vi "HIOKI PW3390 Conf Current.vi"(0 "VISA Resource":refnum<visa-resource-name>, 1 "Set/Query (F: Set)":bool, 2 "CH (1)":i32=1 min=1 max=4, 5 "Auto (F: OFF)":bool, 7 "Range (18: 500A)":T1(ring)=enum."500", 9 "I rect (F: RMS)":bool, 11 "error in (no error)":errorcluster, 12 "OPC query (T: ON)":bool=TRUE, 13 "Error Out (F: Off)":bool) -> (4 "VISA Resource out":refnum<visa-resource-name>, 6 "Auto out":bool, 8 "Range out":dbl=500.0 format="%.1f", 10 "I rect out":bool, 15 "error out":errorcluster)   [LabVIEW 2009]
doc: "Set/Query\n Set: Send the setting commands for the device.\n Query: Query the setting of the device.\n\nAuto\n Sets the current range to AutoRange.\n\nRange\n Sets the current range. Valid when the AutoRange is OFF.\n\nI rect\n Sets the Electric Current Rectification Method to RMS/MEAN.\n\n<B>Note</B>\n Depending on the measurement line combination (for 1P3W and above), the current AutoRange settings of other channels in the combination may be changed too."
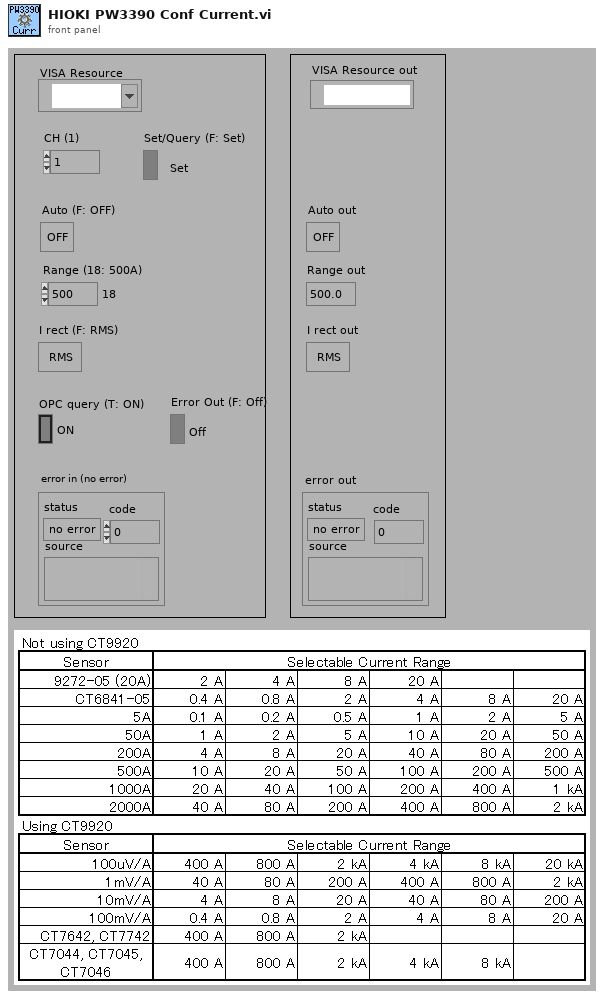
[diagram p1: front panel]
types:
  T1 = enum16{"0.1", "0.2", "0.4", "0.5", "0.8", "1", "2", "4", "5", "8", "10", "20", "40", "50", "80", "100", "200", "400", "500", "800", "1000", "2000", "4000", "8000", "20000"}
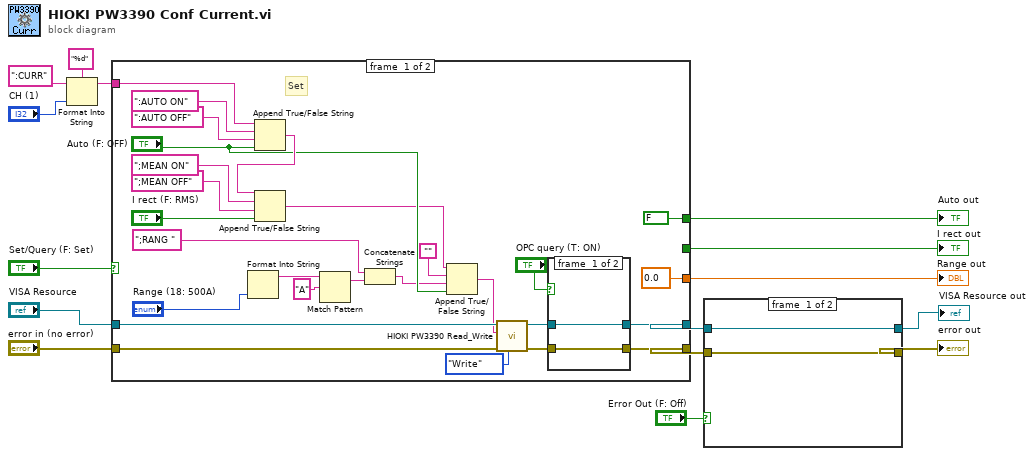
[diagram p0: block diagram]
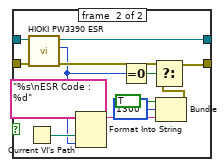
[diagram p2: hidden frame]
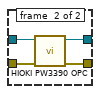
[diagram p3: hidden frame]
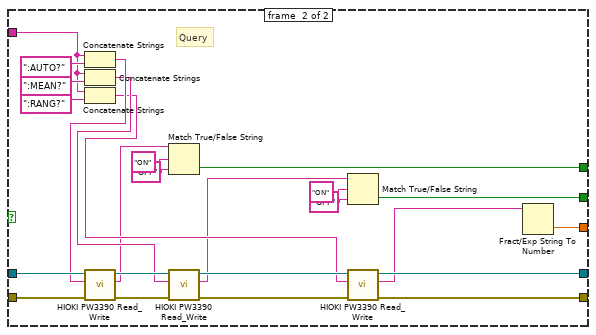
[diagram p4: hidden frame]
diagram:
  n1 = Format Into String(format string="%d", initial string=":CURR", "CH (1)") -> (resulting string=w10:string)  [unwired: 1 in, 1 out]
  n2 = case shown="FALSE" "Set/Query (F: Set)" {
    tunnel: "error in (no error)" -> [w29 w57]
    tunnel: [w22 w56] -> w5
    tunnel: "VISA Resource" -> [w30 w58]
    tunnel: [w23 w55] -> w4
    tunnel: w10 -> [w38 w69]
    tunnel: [0.0 w72] -> w9
    tunnel: [w41 w64] -> w8
    tunnel: [w41 w63] -> w7
    frame #0 {
      w41 = FALSE
      # "Set"
      n3 = Format Into String("Range (18: 500A)") -> (resulting string=w21:string)  [unwired: 3 in, 1 out]
      n4 = Append True/False String(1:"Auto (F: OFF)", 2:":AUTO OFF", 3:":AUTO ON", 4:w38) -> (0:w34:string)
      n5 = Append True/False String(1:"I rect (F: RMS)", 2:";MEAN OFF", 3:";MEAN ON", 4:w34) -> (0:w32:string)
      n6 = Match Pattern(string=w21, regular expression="A") -> (before substring=w18:string)  [unwired: 1 in, 3 out]
      n7 = Concatenate Strings(";RANG ", w18) -> (w16:string)
      n8 = Append True/False String(1:"Auto (F: OFF)", 2:w16, 3:"", 4:w32) -> (0:w28:string)
      n9 = call <instrlib>:"HIOKI PW3390 Read_Write.vi"("Read/Write"=enum16{"Read", "Write"}."Write", "error in (no error)"=w29, "data in"=w28, "VISA Resource"=w30) -> ("error out"=w24:errorcluster, "VISA Resource out"=w25:refnum<visa-resource-name>)  [unwired: 5 in, 1 out]
      n10 = case shown="TRUE" "OPC query (T: ON)" {
        tunnel: [w44 w48] -> w23
        tunnel: [w43 w47] -> w22
        tunnel: w25 -> [w44 w46]
        tunnel: w24 -> [w43 w45]
        frame #0 {
        }
        frame #1 {
          n11 = call <instrlib>:"HIOKI PW3390 OPC.vi"("error in (no error)"=w45, "VISA Resource"=w46) -> ("error out"=w47:errorcluster, "VISA Resource out"=w48:refnum<visa-resource-name>)  [unwired: 7 in, 1 out]
        }
      }
    }
    frame #1 {
      # "Query"
      n12 = Concatenate Strings(w69, ":AUTO?") -> (w54:string)
      n13 = Concatenate Strings(w69, ":MEAN?") -> (w53:string)
      n14 = Concatenate Strings(w69, ":RANG?") -> (w52:string)
      n15 = call <instrlib>:"HIOKI PW3390 Read_Write.vi"("error in (no error)"=w57, "data in"=w54, "VISA Resource"=w58) -> ("error out"=w61:errorcluster, "data out"=w51:string, "VISA Resource out"=w59:refnum<visa-resource-name>)  [unwired: 6 in]
      n16 = Match True/False String(2:"OFF", 3:"ON", 4:w51) -> (0:w64:bool)  [unwired: 1 out]
      n17 = call <instrlib>:"HIOKI PW3390 Read_Write.vi"("error in (no error)"=w61, "data in"=w53, "VISA Resource"=w59) -> ("error out"=w62:errorcluster, "data out"=w50:string, "VISA Resource out"=w60:refnum<visa-resource-name>)  [unwired: 6 in]
      n18 = Match True/False String(2:"OFF", 3:"ON", 4:w50) -> (0:w63:bool)  [unwired: 1 out]
      n19 = call <instrlib>:"HIOKI PW3390 Read_Write.vi"("error in (no error)"=w62, "data in"=w52, "VISA Resource"=w60) -> ("error out"=w56:errorcluster, "data out"=w49:string, "VISA Resource out"=w55:refnum<visa-resource-name>)  [unwired: 6 in]
      n20 = Fract/Exp String To Number(string=w49) -> (number=w72:dbl)  [unwired: 3 in, 1 out]
    }
  }
  "Auto out" <- w8
  "I rect out" <- w7
  "Range out" <- w9
  n21 = case shown="TRUE" "Error Out (F: Off)" {
    tunnel: w4 -> [w75 w88]
    tunnel: w5 -> [w74 w87]
    tunnel: [w74 w77] -> w3
    tunnel: [w75 w86] -> w1
    frame #0 {
    }
    frame #1 {
      n22 = Current VI's Path() -> (path=w84:path)
      n23 = call <instrlib>:"HIOKI PW3390 ESR.vi"("error in (no error)"=w87, "VISA Resource"=w88) -> ("error out"=w78:errorcluster, "Output Value"=w76:u8, "VISA Resource out"=w86:refnum<visa-resource-name>)  [unwired: 6 in, 1 out]
      n24 = Format Into String(format string="%s\nESR Code : %d", w84, w76) -> (resulting string=w80:string)  [unwired: 2 in, 1 out]
      n25 = Equal To 0?(x=w76) -> (x = 0?=w85:bool)
      n26 = Bundle("status"=TRUE, "code"=1300, w80) -> (w79:cluster{"status":bool, "code":i32, string})  [unwired: 1 in]
      n27 = Select(t=w78, s=w85, f=w79) -> (s? t:f=w77:errorcluster)
    }
  }
  "error out" <- w3
  "VISA Resource out" <- w1
